vi "W7X1DPut.vi"(4 "dimensions":i64[](array[numeric])=[1428413878000000000, -1], 7 "Unit":string="s", 10 "SigJSONbuffer":string, 11 "SigLabel":string="MTau") -> ()   [LabVIEW 2014]
uses:
  <vilib>/httpClient/POSTBuffer.vi
  <vilib>/httpClient/LabVIEWHTTPClient.lvlib
panel:
  in  "values":T1(array[cluster])=[{"chanDescs"=[{"name"="E_Chan_1", "active"=1, "physicalQuantity"={"type"="A"}}, {"name"="E_Chan_2", "active"=1, "physicalQuantity"={"type"="A"}}, {"name"="E_Chan_3", "active"=1, "physicalQuantity"={"type"="A"}}, {"name"="E_Chan_4", "active"=1, "physicalQuantity"={"type"="A"}}, {"name"="E_Chan_5", "active"=1, "physicalQuantity"={"type"="A"}}, {"name"="E_Chan_6", "active"=1, "physicalQuantity"={"type"="A"}}, {"name"="E_Chan_7", "active"=1, "physicalQuantity"={"type"="A"}}, {"name"="E_Chan_8", "active"=1, "physicalQuantity"={"type"="A"}}, {"name"="E_Chan_9", "active"=1, "physicalQuantity"={"type"="A"}}, {"name"="E_Chan_10", "active"=1, "physicalQuantity"={"type"="A"}}, {"name"="E_Chan_11", "active"=1, "physicalQuantity"={"type"="A"}}, {"name"="E_Chan_12", "active"=1, "physicalQuantity"={"type"="A"}}, {"name"="E_Chan_13", "active"=1, "physicalQuantity"={"type"="A"}}, {"name"="E_Chan_14", "active"=1, "physicalQuantity"={"type"="A"}}, {"name"="E_Chan_15", "active"=1, "physicalQuantity"={"type"="A"}}, {"name"="E_Chan_16", "active"=1, "physicalQuantity"={"type"="A"}}, {"name"="E_Chan_17", "active"=1, "physicalQuantity"={"type"="A"}}, {"name"="E_Chan_18", "active"=1, "physicalQuantity"={"type"="A"}}, {"name"="E_Chan_19", "active"=1, "physicalQuantity"={"type"="A"}}, {"name"="E_Chan_20", "active"=1, "physicalQuantity"={"type"="A"}}, {"name"="E_Chan_21", "active"=1, "physicalQuantity"={"type"="A"}}, {"name"="E_Chan_22", "active"=1, "physicalQuantity"={"type"="A"}}, {"name"="E_Chan_23", "active"=1, "physicalQuantity"={"type"="A"}}, {"name"="E_Chan_24", "active"=1, "physicalQuantity"={"type"="A"}}, {"name"="E_Chan_25", "active"=1, "physicalQuantity"={"type"="A"}}, {"name"="E_Chan_26", "active"=1, "physicalQuantity"={"type"="A"}}, {"name"="E_Chan_27", "active"=1, "physicalQuantity"={"type"="A"}}, {"name"="E_Chan_28", "active"=1, "physicalQuantity"={"type"="A"}}, {"name"="E_Chan_29", "active"=1, "physicalQuantity"={"type"="A"}}, {"name"="E_Chan_30", "active"=1, "physicalQuantity"={"type"="A"}}, {"name"="E_Chan_31", "active"=1, "physicalQuantity"={"type"="A"}}, {"name"="E_Chan_32", "active"=1, "physicalQuantity"={"type"="A"}}, {"name"="E_Chan_33", "active"=1, "physicalQuantity"={"type"="A"}}, {"name"="E_Chan_34", "active"=1, "physicalQuantity"={"type"="A"}}, {"name"="E_Chan_35", "active"=1, "physicalQuantity"={"type"="A"}}, {"name"="E_Chan_36", "active"=1, "physicalQuantity"={"type"="A"}}, {"name"="E_Chan_37", "active"=1, "physicalQuantity"={"type"="A"}}, {"name"="E_Chan_38", "active"=1, "physicalQuantity"={"type"="A"}}, {"name"="E_Chan_39", "active"=1, "physicalQuantity"={"type"="A"}}, {"name"="E_Chan_40", "active"=1, "physicalQuantity"={"type"="A"}}, {"name"="E_Chan_41", "active"=1, "physicalQuantity"={"type"="A"}}, {"name"="E_Chan_42", "active"=1, "physicalQuantity"={"type"="A"}}, {"name"="E_Chan_43", "active"=1, "physicalQuantity"={"type"="A"}}, {"name"="E_Chan_44", "active"=1, "physicalQuantity"={"type"="A"}}, {"name"="E_Chan_45", "active"=1, "physicalQuantity"={"type"="A"}}, {"name"="E_Chan_46", "active"=1, "physicalQuantity"={"type"="A"}}, {"name"="E_Chan_47", "active"=1, "physicalQuantity"={"type"="A"}}, {"name"="E_Chan_48", "active"=1, "physicalQuantity"={"type"="A"}}, {"name"="E_Chan_49", "active"=1, "physicalQuantity"={"type"="A"}}, {"name"="E_Chan_50", "active"=1, "physicalQuantity"={"type"="A"}}, {"name"="E_Chan_51", "active"=1, "physicalQuantity"={"type"="A"}}, {"name"="E_Chan_52", "active"=1, "physicalQuantity"={"type"="A"}}, {"name"="E_Chan_53", "active"=1, "physicalQuantity"={"type"="A"}}, {"name"="E_Chan_54", "active"=1, "physicalQuantity"={"type"="A"}}, {"name"="E_Chan_55", "active"=1, "physicalQuantity"={"type"="A"}}, {"name"="E_Chan_56", "active"=1, "physicalQuantity"={"type"="A"}}, {"name"="E_Chan_57", "active"=1, "physicalQuantity"={"type"="A"}}, {"name"="E_Chan_58", "active"=1, "physicalQuantity"={"type"="A"}}, {"name"="E_Chan_59", "active"=1, "physicalQuantity"={"type"="A"}}, {"name"="E_Chan_60", "active"=1, "physicalQuantity"={"type"="A"}}, {"name"="E_Chan_61", "active"=1, "physicalQuantity"={"type"="A"}}, {"name"="E_Chan_62", "active"=1, "physicalQuantity"={"type"="A"}}, {"name"="E_Chan_63", "active"=1, "physicalQuantity"={"type"="A"}}, {"name"="E_Chan_64", "active"=1, "physicalQuantity"={"type"="A"}}, {"name"="E_Chan_65", "active"=1, "physicalQuantity"={"type"="A"}}, {"name"="E_Chan_66", "active"=1, "physicalQuantity"={"type"="A"}}, {"name"="E_Chan_67", "active"=1, "physicalQuantity"={"type"="A"}}, {"name"="E_Chan_68", "active"=1, "physicalQuantity"={"type"="A"}}, {"name"="E_Chan_69", "active"=1, "physicalQuantity"={"type"="A"}}, {"name"="E_Chan_70", "active"=1, "physicalQuantity"={"type"="A"}}, {"name"="E_Chan_71", "active"=1, "physicalQuantity"={"type"="A"}}, {"name"="E_Chan_72", "active"=1, "physicalQuantity"={"type"="A"}}, {"name"="E_Chan_73", "active"=1, "physicalQuantity"={"type"="A"}}, {"name"="E_Chan_74", "active"=1, "physicalQuantity"={"type"="A"}}, {"name"="E_Chan_75", "active"=1, "physicalQuantity"={"type"="A"}}, {"name"="E_Chan_76", "active"=1, "physicalQuantity"={"type"="A"}}, {"name"="E_Chan_77", "active"=1, "physicalQuantity"={"type"="A"}}, {"name"="E_Chan_78", "active"=1, "physicalQuantity"={"type"="A"}}, {"name"="E_Chan_79", "active"=1, "physicalQuantity"={"type"="A"}}, {"name"="E_Chan_80", "active"=1, "physicalQuantity"={"type"="A"}}, {"name"="E_Chan_81", "active"=1, "physicalQuantity"={"type"="A"}}, {"name"="E_Chan_82", "active"=1, "physicalQuantity"={"type"="A"}}, {"name"="E_Chan_83", "active"=1, "physicalQuantity"={"type"="A"}}, {"name"="E_Chan_84", "active"=1, "physicalQuantity"={"type"="A"}}, {"name"="E_Chan_85", "active"=1, "physicalQuantity"={"type"="A"}}, {"name"="E_Chan_86", "active"=1, "physicalQuantity"={"type"="A"}}, {"name"="E_Chan_87", "active"=1, "physicalQuantity"={"type"="A"}}, {"name"="E_Chan_88", "active"=1, "physicalQuantity"={"type"="A"}}, {"name"="E_Chan_89", "active"=1, "physicalQuantity"={"type"="A"}}, {"name"="E_Chan_90", "active"=1, "physicalQuantity"={"type"="A"}}, {"name"="E_Chan_91", "active"=1, "physicalQuantity"={"type"="A"}}, {"name"="E_Chan_92", "active"=1, "physicalQuantity"={"type"="A"}}, {"name"="E_Chan_93", "active"=1, "physicalQuantity"={"type"="A"}}, {"name"="E_Chan_94", "active"=1, "physicalQuantity"={"type"="A"}}, {"name"="E_Chan_95", "active"=1, "physicalQuantity"={"type"="A"}}, {"name"="E_Chan_96", "active"=1, "physicalQuantity"={"type"="A"}}, {"name"="E_Chan_97", "active"=1, "physicalQuantity"={"type"="A"}}, {"name"="E_Chan_98", "active"=1, "physicalQuantity"={"type"="A"}}, {"name"="E_Chan_99", "active"=1, "physicalQuantity"={"type"="A"}}, {"name"="E_Chan_100", "active"=1, "physicalQuantity"={"type"="A"}}, {"name"="E_Chan_101", "active"=1, "physicalQuantity"={"type"="A"}}, {"name"="E_Chan_102", "active"=1, "physicalQuantity"={"type"="A"}}, {"name"="E_Chan_103", "active"=1, "physicalQuantity"={"type"="A"}}, {"name"="E_Chan_104", "active"=1, "physicalQuantity"={"type"="A"}}, {"name"="E_Chan_105", "active"=1, "physicalQuantity"={"type"="A"}}, {"name"="E_Chan_106", "active"=1, "physicalQuantity"={"type"="A"}}, {"name"="E_Chan_107", "active"=1, "physicalQuantity"={"type"="A"}}, {"name"="E_Chan_108", "active"=1, "physicalQuantity"={"type"="A"}}, {"name"="E_Chan_109", "active"=1, "physicalQuantity"={"type"="A"}}, {"name"="E_Chan_110", "active"=1, "physicalQuantity"={"type"="A"}}, {"name"="E_Chan_111", "active"=1, "physicalQuantity"={"type"="A"}}, {"name"="E_Chan_112", "active"=1, "physicalQuantity"={"type"="A"}}, {"name"="E_Chan_113", "active"=1, "physicalQuantity"={"type"="A"}}, {"name"="E_Chan_114", "active"=1, "physicalQuantity"={"type"="A"}}, {"name"="E_Chan_115", "active"=1, "physicalQuantity"={"type"="A"}}, {"name"="E_Chan_116", "active"=1, "physicalQuantity"={"type"="A"}}, {"name"="E_Chan_117", "active"=1, "physicalQuantity"={"type"="A"}}, {"name"="E_Chan_118", "active"=1, "physicalQuantity"={"type"="A"}}, {"name"="E_Chan_119", "active"=1, "physicalQuantity"={"type"="A"}}, {"name"="E_Chan_120", "active"=1, "physicalQuantity"={"type"="A"}}, {"name"="E_Chan_121", "active"=1, "physicalQuantity"={"type"="A"}}, {"name"="E_Chan_122", "active"=1, "physicalQuantity"={"type"="A"}}, {"name"="E_Chan_123", "active"=1, "physicalQuantity"={"type"="A"}}, {"name"="E_Chan_124", "active"=1, "physicalQuantity"={"type"="A"}}, {"name"="E_Chan_125", "active"=1, "physicalQuantity"={"type"="A"}}, {"name"="E_Chan_126", "active"=1, "physicalQuantity"={"type"="A"}}, {"name"="E_Chan_127", "active"=1, "physicalQuantity"={"type"="A"}}, {"name"="E_Chan_128", "active"=1, "physicalQuantity"={"type"="A"}}], "detector"="Au_Kapton", "NChannels"=128, "ADCBits"=16, "CalStep1 (V)"="2.5", "CalStep2 (V)"="3.7"}]
  in  "?":T2
  in  "chanDescs2D":T3(array[cluster])=[[{"name"="HBCm_U30_01", "active"=1, "physicalQuantity"={"type"="A"}}, {"name"="HBCm_U30_02", "active"=1, "physicalQuantity"={"type"="A"}}, {"name"="HBCm_U30_03", "active"=1, "physicalQuantity"={"type"="A"}}, {"name"="HBCm_U30_04", "active"=1, "physicalQuantity"={"type"="A"}}, {"name"="HBCm_U30_05", "active"=1, "physicalQuantity"={"type"="A"}}, {"name"="HBCm_U30_06", "active"=1, "physicalQuantity"={"type"="A"}}, {"name"="HBCm_U30_07", "active"=1, "physicalQuantity"={"type"="A"}}, {"name"="HBCm_U30_08", "active"=1, "physicalQuantity"={"type"="A"}}, {"name"="HBCm_U30_09", "active"=1, "physicalQuantity"={"type"="A"}}, {"name"="HBCm_U30_10", "active"=1, "physicalQuantity"={"type"="A"}}, {"name"="HBCm_U30_11", "active"=1, "physicalQuantity"={"type"="A"}}, {"name"="HBCm_U30_12", "active"=1, "physicalQuantity"={"type"="A"}}, {"name"="HBCm_U30_013", "active"=1, "physicalQuantity"={"type"="A"}}, {"name"="HBCm_U30_14", "active"=1, "physicalQuantity"={"type"="A"}}, {"name"="HBCm_U30_15", "active"=1, "physicalQuantity"={"type"="A"}}, {"name"="HBCm_U30_16", "active"=1, "physicalQuantity"={"type"="A"}}, {"name"="HBCm_U30_17", "active"=1, "physicalQuantity"={"type"="A"}}, {"name"="HBCm_U30_18", "active"=1, "physicalQuantity"={"type"="A"}}, {"name"="HBCm_U30_19", "active"=1, "physicalQuantity"={"type"="A"}}, {"name"="HBCm_U30_20", "active"=1, "physicalQuantity"={"type"="A"}}, {"name"="HBCm_U30_21", "active"=1, "physicalQuantity"={"type"="A"}}, {"name"="HBCm_U30_22", "active"=1, "physicalQuantity"={"type"="A"}}, {"name"="HBCm_U30_23", "active"=1, "physicalQuantity"={"type"="A"}}, {"name"="HBCm_U30_24", "active"=1, "physicalQuantity"={"type"="A"}}, {"name"="HBCm_U30_25", "active"=1, "physicalQuantity"={"type"="A"}}, {"name"="HBCm_U30_26", "active"=1, "physicalQuantity"={"type"="A"}}, {"name"="HBCm_U30_27", "active"=1, "physicalQuantity"={"type"="A"}}, {"name"="HBCm_U30_28", "active"=1, "physicalQuantity"={"type"="A"}}, {"name"="HBCm_U30_29", "active"=1, "physicalQuantity"={"type"="A"}}, {"name"="HBCm_U30_30", "active"=1, "physicalQuantity"={"type"="A"}}, {"name"="HBCm_U30_31", "active"=1, "physicalQuantity"={"type"="A"}}, {"name"="HBCm_U30_32", "active"=1, "physicalQuantity"={"type"="A"}}, {"name"="VBCm_V21_01", "active"=1, "physicalQuantity"={"type"="A"}}, {"name"="VBCm_V21_02", "active"=1, "physicalQuantity"={"type"="A"}}, {"name"="VBCm_V21_03", "active"=1, "physicalQuantity"={"type"="A"}}, {"name"="VBCm_V21_04", "active"=1, "physicalQuantity"={"type"="A"}}, {"name"="VBCm_V21_05", "active"=1, "physicalQuantity"={"type"="A"}}, {"name"="VBCm_V21_06", "active"=1, "physicalQuantity"={"type"="A"}}, {"name"="VBCm_V21_07", "active"=1, "physicalQuantity"={"type"="A"}}, {"name"="VBCm_V21_08", "active"=1, "physicalQuantity"={"type"="A"}}, {"name"="VBCm_V21_09", "active"=1, "physicalQuantity"={"type"="A"}}, {"name"="VBCm_V21_10", "active"=1, "physicalQuantity"={"type"="A"}}, {"name"="VBCm_V21_11", "active"=1, "physicalQuantity"={"type"="A"}}, {"name"="VBCm_V21_12", "active"=1, "physicalQuantity"={"type"="A"}}, {"name"="VBCm_V21_13", "active"=1, "physicalQuantity"={"type"="A"}}, {"name"="VBCm_V21_14", "active"=1, "physicalQuantity"={"type"="A"}}, {"name"="VBCm_V21_15", "active"=1, "physicalQuantity"={"type"="A"}}, {"name"="VBCm_V21_16", "active"=1, "physicalQuantity"={"type"="A"}}, {"name"="VBCm_V21_17", "active"=1, "physicalQuantity"={"type"="A"}}, {"name"="VBCm_V21_18", "active"=1, "physicalQuantity"={"type"="A"}}, {"name"="VBCm_V21_19", "active"=1, "physicalQuantity"={"type"="A"}}, {"name"="VBCm_V21_20", "active"=1, "physicalQuantity"={"type"="A"}}, {"name"="VBCm_V21_21", "active"=1, "physicalQuantity"={"type"="A"}}, {"name"="VBCm_V21_22", "active"=1, "physicalQuantity"={"type"="A"}}, {"name"="VBCm_V21_23", "active"=1, "physicalQuantity"={"type"="A"}}, {"name"="VBCm_V21_24", "active"=1, "physicalQuantity"={"type"="A"}}, {"name"="VBCm_V21_25", "active"=1, "physicalQuantity"={"type"="A"}}, {"name"="VBCm_V21_26", "active"=1, "physicalQuantity"={"type"="A"}}, {"name"="VBCm_V21_27", "active"=1, "physicalQuantity"={"type"="A"}}, {"name"="VBCm_V21_28", "active"=1, "physicalQuantity"={"type"="A"}}, {"name"="VBCm_V21_29", "active"=1, "physicalQuantity"={"type"="A"}}, {"name"="VBCm_V21_30", "active"=1, "physicalQuantity"={"type"="A"}}, {"name"="VBCm_V21_31", "active"=1, "physicalQuantity"={"type"="A"}}, {"name"="VBCm_V21_32", "active"=1, "physicalQuantity"={"type"="A"}}, {"name"="VBCm_V21_33", "active"=1, "physicalQuantity"={"type"="A"}}, {"name"="VBCm_V21_34", "active"=1, "physicalQuantity"={"type"="A"}}, {"name"="VBCm_V21_35", "active"=1, "physicalQuantity"={"type"="A"}}, {"name"="VBCm_V21_36", "active"=1, "physicalQuantity"={"type"="A"}}, {"name"="VBCm_V21_37", "active"=1, "physicalQuantity"={"type"="A"}}, {"name"="VBCm_V21_38", "active"=1, "physicalQuantity"={"type"="A"}}, {"name"="VBCm_V21_39", "active"=1, "physicalQuantity"={"type"="A"}}, {"name"="VBCm_V21_40", "active"=1, "physicalQuantity"={"type"="A"}}, {"name"="VBCs_V21_01", "active"=1, "physicalQuantity"={"type"="A"}}, {"name"="VBCs_V21_02", "active"=1, "physicalQuantity"={"type"="A"}}, {"name"="VBCs_V21_03", "active"=1, "physicalQuantity"={"type"="A"}}, {"name"="VBCs_V21_04", "active"=1, "physicalQuantity"={"type"="A"}}, {"name"="VBCs_V21_05", "active"=1, "physicalQuantity"={"type"="A"}}, {"name"="VBCs_V21_06", "active"=1, "physicalQuantity"={"type"="A"}}, {"name"="VBCs_V21_07", "active"=1, "physicalQuantity"={"type"="A"}}, {"name"="VBCs_V21_08", "active"=1, "physicalQuantity"={"type"="A"}}, {"name"="HBCs_U30_01", "active"=1, "physicalQuantity"={"type"="A"}}, {"name"="HBCs_U30_02", "active"=1, "physicalQuantity"={"type"="A"}}, {"name"="HBCs_U30_03", "active"=1, "physicalQuantity"={"type"="A"}}, {"name"="HBCs_U30_04", "active"=1, "physicalQuantity"={"type"="A"}}, {"name"="HBCs_U30_05", "active"=1, "physicalQuantity"={"type"="A"}}, {"name"="HBCs_U30_06", "active"=1, "physicalQuantity"={"type"="A"}}, {"name"="HBCs_U30_07", "active"=1, "physicalQuantity"={"type"="A"}}, {"name"="HBCs_U30_08", "active"=1, "physicalQuantity"={"type"="A"}}, {"name"="HBCs_U30_09", "active"=1, "physicalQuantity"={"type"="A"}}, {"name"="HBCs_U30_10", "active"=1, "physicalQuantity"={"type"="A"}}, {"name"="HBCs_U30_11", "active"=1, "physicalQuantity"={"type"="A"}}, {"name"="HBCs_U30_12", "active"=1, "physicalQuantity"={"type"="A"}}, {"name"="HBCs_U30_13", "active"=1, "physicalQuantity"={"type"="A"}}, {"name"="HBCs_U30_14", "active"=1, "physicalQuantity"={"type"="A"}}, {"name"="HBCs_U30_15", "active"=1, "physicalQuantity"={"type"="A"}}, {"name"="", "active"=1, "physicalQuantity"={"type"=""}}]]
  out "JSON string":string
  out "body":string
  out "headers":string
  out "body Parlog":string
  out "headers parms":string
  out "Parlog error out":errorcluster
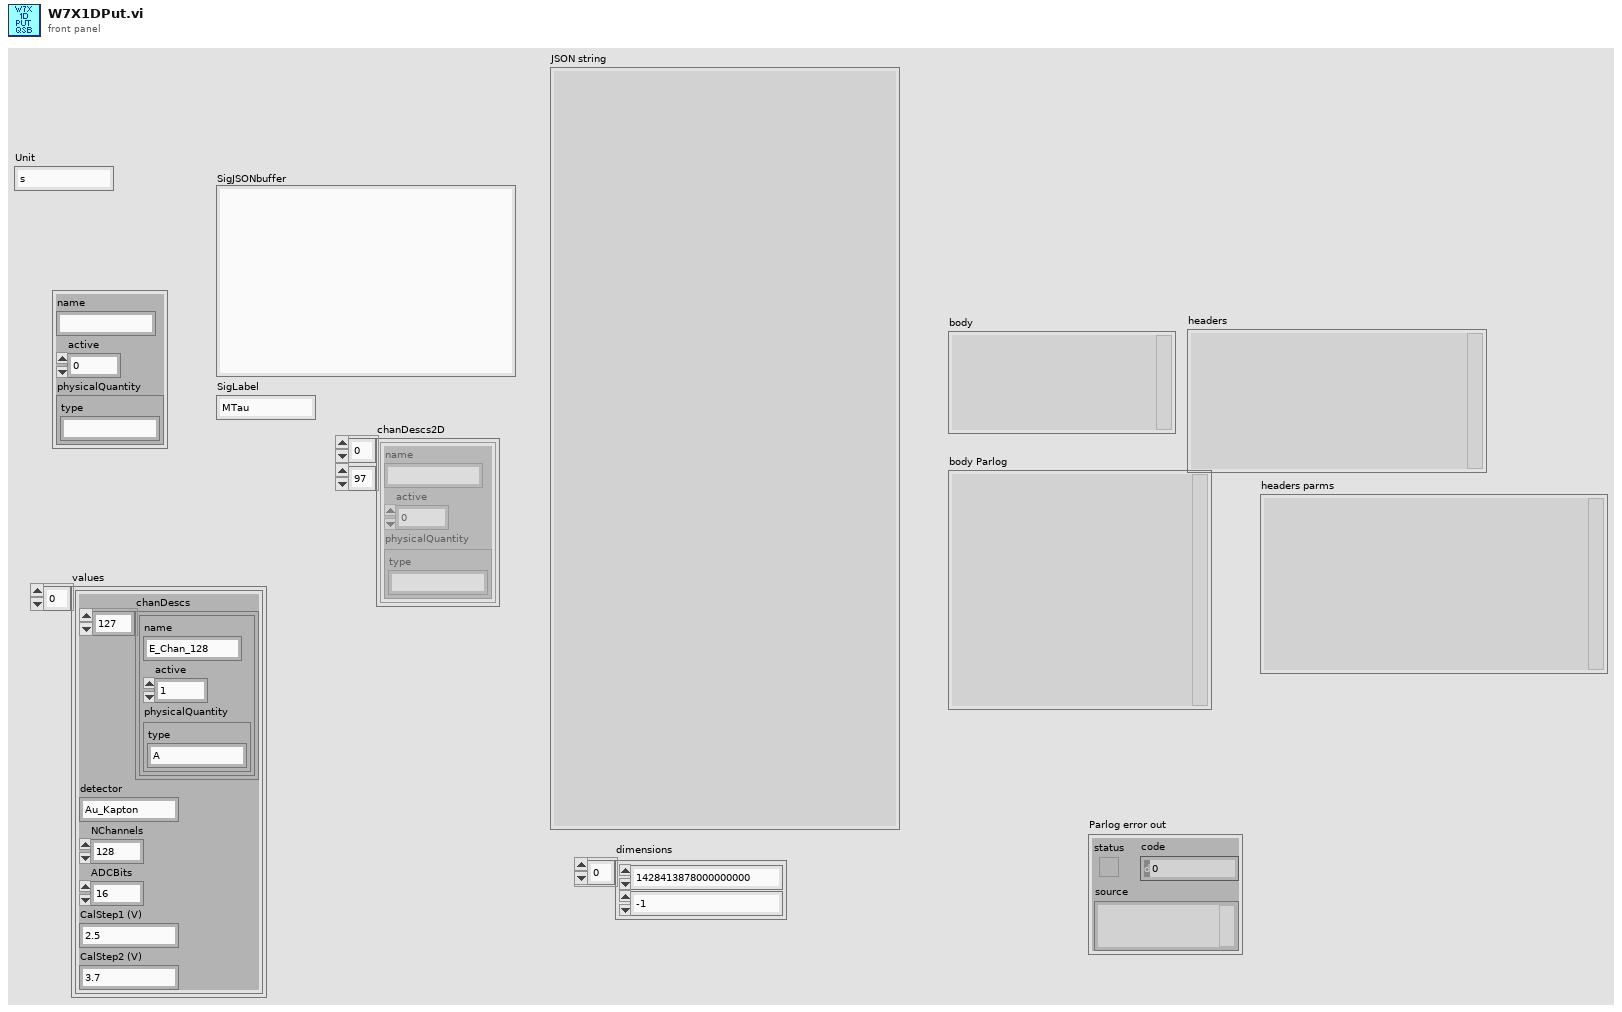
[diagram p1: front panel]
types:
  T1 = cluster{"chanDescs":cluster{"name":string, "active":i32, "physicalQuantity":cluster{"type":string}}[], "detector":string, "NChannels":u16, "ADCBits":u16, "CalStep1 (V)":string, "CalStep2 (V)":string}[]
  T2 = cluster{"name":string, "active":i32, "physicalQuantity":cluster{"type":string}}
  T3 = cluster{"name":string, "active":i32, "physicalQuantity":cluster{"type":string}}[][]
  T4 = cluster{"chanDescs":cluster{"name":string, "active":i32, "physicalQuantity":cluster{"type":string}}[], "detector":string, "NChannels":u16, "ADCBits":u16, "CalStep1 (V)":string, "CalStep2 (V)":string}
  T5 = cluster{"name":string, "active":i32, "physicalQuantity":cluster{"type":string}}[]
  T6 = typedef "LabVIEWHTTPClient.lvlib/ClientHandle.ctl" = refnum<k1>
  T7 = cluster{"label":string, "values":cluster{"chanDescs":cluster{"name":string, "active":i32, "physicalQuantity":cluster{"type":string}}[], "detector":string, "NChannels":u16, "ADCBits":u16, "CalStep1 (V)":string, "CalStep2 (V)":string}[], "dimensions":i64[]}
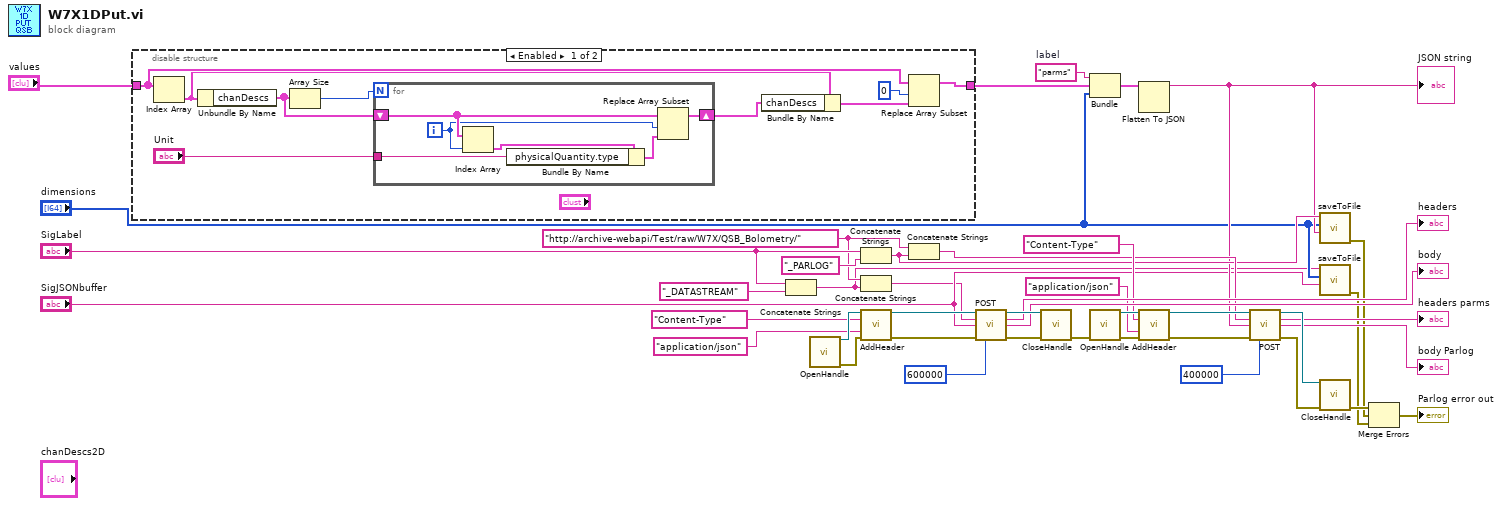
[diagram p0: block diagram]
diagram:
  w30 = "parms"  # label
  w5 = "http://archive-webapi/Test/raw/W7X/QSB_Bolometry/" ("url")
  n1 = disable-structure shown="Enabled" {
    disable-tunnel: "values" -> [w51 w58]
    disable-tunnel: [w50 w58] -> w28
    frame Enabled {
      n2 = Index Array(array=w51) -> (element=w48:T4)  [unwired: 1 in]
      n3 = Unbundle By Name(w48) -> ("chanDescs"=w44:T5)
      n4 = Array Size(array=w44) -> (size(s)=w43:i32)
      n5 = for {
        N: w43 -> [_]
        tunnel: "Unit" -> [w57]
        shift-right: [w53] -> w45
        shift-left: w44 -> [w55]
        i -> [w52]
        n6 = Index Array(array=w55, index=w52) -> (element=w56:T2)
        n7 = Bundle By Name(cluster=w56, "physicalQuantity.type"=w57) -> (w54:T2)
        n8 = Replace Array Subset(array=w55, new element=w54, index=w52) -> (w53:T5)
      }
      n9 = Bundle By Name(cluster=w48, "chanDescs"=w45) -> (w47:T4)
      n10 = Replace Array Subset(array=w51, new element=w47, index=0) -> (w50:T1)
    }
    frame Disabled {
    }
  }
  n11 = Concatenate Strings("SigLabel", "_DATASTREAM" ("string")) -> (w4:string)
  n12 = call <vilib>:"OpenHandle.vi"() -> ("client handle out"=w39:T6, "error out"=w38:errorcluster)  [unwired: 14 in]
  n13 = Concatenate Strings("SigLabel", "_PARLOG" ("replace string (\"\")")) -> (w10:string)
  n14 = Concatenate Strings(w5, w4) -> (w6:string)
  n15 = call <vilib>:"AddHeader.vi"("client handle"=w39, "header"="Content-Type", "value"="application/json", "error in (no error)"=w38) -> ("client handle out"=w37:T6, "error out"=w36:errorcluster)  [unwired: 10 in]
  n16 = Concatenate Strings(w5, w10) -> (w11:string)
  n17 = call-poly <vilib>:"POST.vi"("client handle"=w37, "url"=w6, "buffer"="SigJSONbuffer", "error in (no error)"=w36, "timeout (10000)"=600000) -> ("client handle out"=w42:T6, "headers"=→"headers":string, "body"=→"body":string, "error out"=w41:errorcluster)  [unwired: 7 in]
  n18 = call <vilib>:"CloseHandle.vi"("client handle"=w42, "error in (no error)"=w41) -> ("error out"=w3:errorcluster)  [unwired: 13 in]
  n19 = Bundle("label"=w30, "values"=w28, "dimensions"="dimensions") -> (w29:T7)  [unwired: 1 in]
  n20 = call <vilib>:"OpenHandle.vi"("error in (no error)"=w3) -> ("client handle out"=w24:T6, "error out"=w23:errorcluster)  [unwired: 13 in]
  n21 = Flatten To JSON(anything=w29) -> (JSON string=w9:string)  [unwired: 2 in, 1 out]
  "JSON string" <- w9
  n22 = call <vilib>:"AddHeader.vi"("client handle"=w24, "header"="Content-Type", "value"="application/json", "error in (no error)"=w23) -> ("client handle out"=w22:T6, "error out"=w21:errorcluster)  [unwired: 10 in]
  n23 = call-poly <vilib>:"POST.vi"("client handle"=w22, "url"=w11, "buffer"=w9, "error in (no error)"=w21, "timeout (10000)"=400000) -> ("client handle out"=w27:T6, "headers"=→"headers parms":string, "body"=→"body Parlog":string, "error out"=w26:errorcluster)  [unwired: 7 in]
  n24 = call "saveToFile.vi"("SigJSONbuffer"=w9, "dimensions"="dimensions", "String"=w10) -> ("error out"=w12:errorcluster)  [unwired: 8 in]
  n25 = call "saveToFile.vi"("SigJSONbuffer"="SigJSONbuffer", "dimensions"="dimensions", "String"=w4) -> ("error out"=w2:errorcluster)  [unwired: 8 in]
  n26 = call <vilib>:"CloseHandle.vi"("client handle"=w27, "error in (no error)"=w26) -> ("error out"=w16:errorcluster)  [unwired: 13 in]
  n27 = Merge Errors(w16, w12, w2) -> (→"Parlog error out":errorcluster)
